vi "Get Log Folder.vi"(5 "Min Free Space (MB)":dbl=50.0, 7 "Max Folders to Check":u32=10, 8 "error in (no error)":errorcluster, 9 "Starting Letter Position":i32=3, 10 "Folder Pattern":string="%s:\\", 11 "Trace Controller in":refnum<class "Trace Controller.lvclass">) -> (0 "error out":errorcluster, 1 "Folder Found?":bool, 2 "Folder":path=path "C:/", 3 "Trace Controller out":refnum<class "Trace Controller.lvclass">)   [LabVIEW 2014, in "Robot Actor Framework.lvlib" / "Trace.lvlib" / "Trace Controller.lvclass"]
uses:
  Trace Controller.lvclass
  Utilities/Utilities.lvlib
panel:
  out "free (bytes)":i64
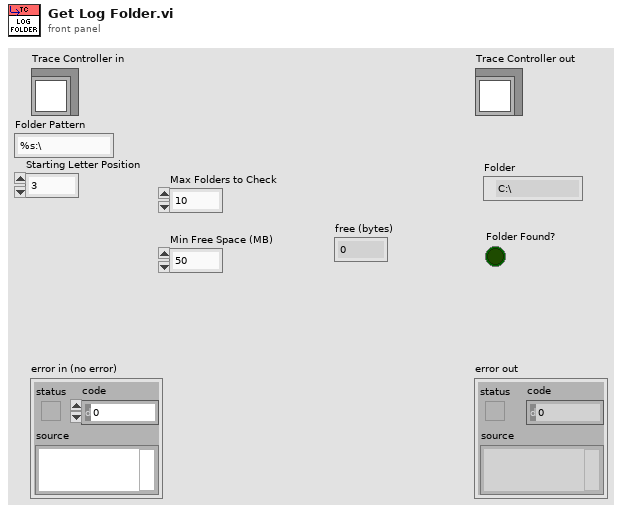
[diagram p1: front panel]
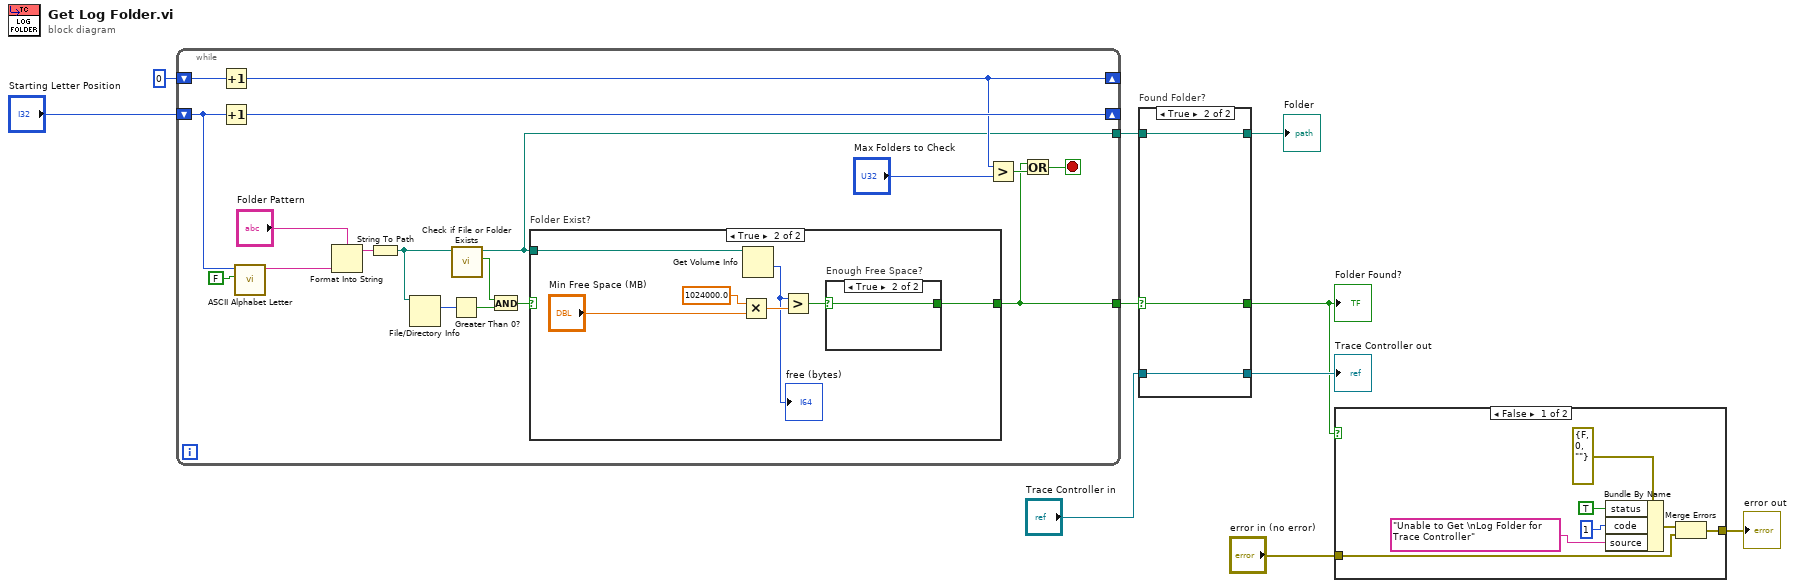
[diagram p0: block diagram]
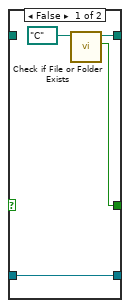
[diagram p3: hidden frame]
diagram:
  n1 = while {
    shift-right: [w24] -> _
    shift-left: "Starting Letter Position" -> [w25]
    shift-right: [w21] -> _
    shift-left: 0 -> [w23]
    tunnel: [w16] -> w9
    tunnel: [w18] -> w10
    stop <- w22 stop-if-true
    n2 = Increment(x=w23) -> (x+1=w21:i32)
    n3 = Increment(x=w25) -> (x+1=w24:i32)
    n4 = call "ASCII Alphabet Letter.vi"("Upper Case?"=FALSE, "Position in Alphabet"=w25) -> ("Letter of Alphabet"=w26:string)  [unwired: 9 in]
    n5 = Format Into String(format string="Folder Pattern", w26) -> (resulting string=w27:string)  [unwired: 2 in, 1 out]
    n6 = String To Path(string=w27) -> (path=w11:path)
    n7 = File/Directory Info(path=w11) -> (size=w12:i64)  [unwired: 1 in, 6 out]
    n8 = Greater Than 0?(x=w12) -> (x > 0?=w13:bool)
    n9 = call <vilib>:"Check if File or Folder Exists.vi"("path"=w11) -> ("file or folder exists?"=w17:bool, "dup path"=w18:path)  [unwired: 8 in, 1 out]
    n10 = And(x=w17, y=w13) -> (x .and. y?=w14:bool)
    n11 = case "Folder Exist?" shown="True" w14 {
      selector: w14 -> [w29 _]
      tunnel: [w29 w32] -> w16
      tunnel: w18 -> [_ w31]
      frame False {
      }
      frame True {
        n12 = Multiply(x=1024000.0, y="Min Free Space (MB)") -> (x*y=w35:dbl)
        n13 = Get Volume Info(11:w31) -> (1:w30:i64)  [unwired: 1 in, 5 out]
        "free (bytes)" <- w30
        n14 = Greater?(x=w30, y=w35) -> (0:w33:bool)
        n15 = case "Enough Free Space?" shown="True" w33 {
          selector: w33 -> [w37 w38]
          tunnel: [w37 w38] -> w32
          frame False {
          }
          frame True {
          }
        }
      }
    }
    n16 = Greater?(x=w21, y="Max Folders to Check") -> (0:w19:bool)
    n17 = Or(x=w16, y=w19) -> (x .or. y?=w22:bool)
  }
  n18 = case "Found Folder?" shown="True" w9 {
    selector: w9 -> [_ w45]
    tunnel: w10 -> [_ w43]
    tunnel: [w39 w45] -> w1
    tunnel: "Trace Controller in" -> [w42 w44]
    tunnel: [w42 w44] -> w5
    tunnel: [w40 w43] -> w2
    frame False {
      n19 = call <vilib>:"Check if File or Folder Exists.vi"("path"=path "C:/") -> ("file or folder exists?"=w39:bool, "dup path"=w40:path)  [unwired: 8 in, 1 out]
    }
    frame True {
    }
  }
  "Trace Controller out" <- w5
  "Folder" <- w2
  "Folder Found?" <- w1
  n20 = case shown="False" w1 {
    tunnel: "error in (no error)" -> [w47 w53]
    tunnel: [w46 w53] -> w3
    frame False {
      n21 = Bundle By Name(cluster=errorcluster {"status"=FALSE, "code"=0, "source"=""} ("error in"), "status"=TRUE, "code"=1, "source"="Unable to Get \nLog Folder for Trace Controller") -> (w48:errorcluster)
      n22 = Merge Errors(w48, w47) -> (w46:errorcluster)
    }
    frame True {
    }
  }
  "error out" <- w3
